vi "Cmag Move to (SubVI).vi"(9 "Instrument":T1 {"Input (1;B)" items=["A", "B"]; "Input (0:A) 325" items=["A", "B"]; "Input (0:A)" items=["A", "B"]; "Heater Output (1:1)" items=["1"=1, "2"=2]}, 10 "字符串":string) -> (0 "错误输出":errorcluster)   [LabVIEW 2019, in "Take Seq.lvlib"]
uses:
  Take Seq.lvlib
  ctl/Instrument.ctl
  <vilib>/NI/Modbus Library/API/Master/Modbus Master.lvclass
  ctl/Instrument Type.ctl
  lib/QDInstrument.dll
  ctl/335 state.ctl
  ctl/limit.ctl
  ctl/9T mag field stauts.ctl
  9T cmag.lvlib
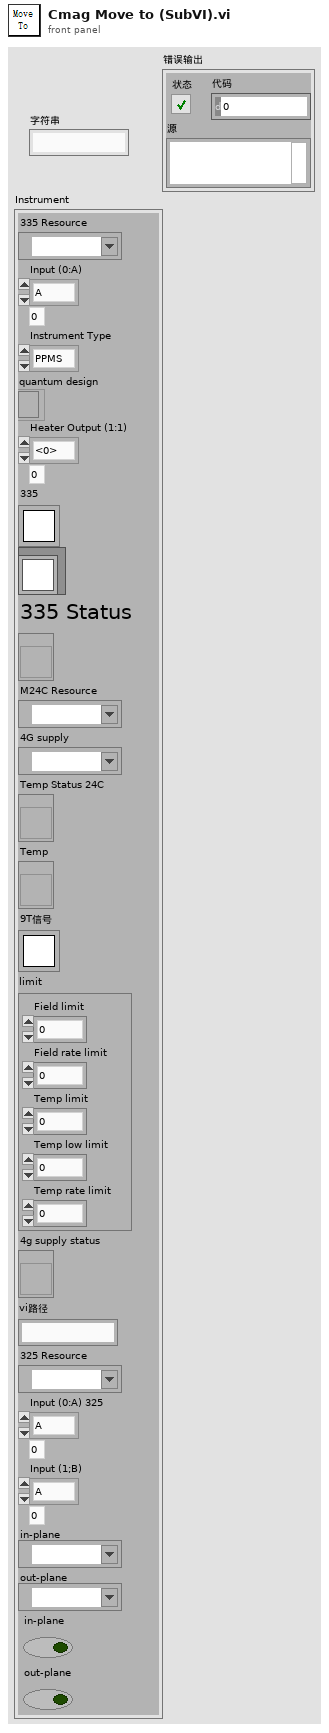
[diagram p1: front panel]
types:
  T1 = typedef "Instrument.ctl" = cluster{"335 Resource":refnum<visa-resource-name>, "Input (0:A)":u16, "Instrument Type":T2, "quantum design":refnum<k24>, "Heater Output (1:1)":u16, "semaphore":T3, "TCP master instance":refnum<class "Modbus Master.lvclass">, "335 Status":refnum<vi>, "M24C Resource":refnum<visa-resource-name>, "4G supply":refnum<visa-resource-name>, "Temp Status 24C":refnum<vi>, "Temp":refnum<vi>, "9T信号":T3, "limit":T4, "4g supply status":refnum<vi>, "vi路径":string, "325 Resource ":refnum<visa-resource-name>, "Input (0:A) 325":u16, "Input (1;B)":u16, "in-plane":refnum<visa-resource-name>, "out-plane":refnum<visa-resource-name>, "in-plane":bool, "out-plane":bool}
  T2 = typedef "Instrument Type.ctl" = enum16{"PPMS", "VersaLab", "DynaCool", "SVSM", "PPMS-Rotate", "Lakeshore335", "9T mag"}
  T3 = typedef "Semaphore RefNum" = refnum<k1>
  T4 = typedef "limit.ctl" = cluster{"Field limit":dbl, "Field rate limit":dbl, "Temp limit":dbl, "Temp low limit":dbl, "Temp rate limit ":dbl}
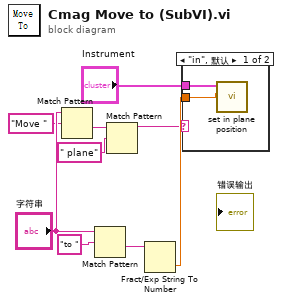
[diagram p0: block diagram]
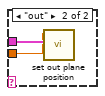
[diagram p2: hidden frame]
diagram:
  n1 = Match Pattern(string="字符串", regular expression="Move " ("正则表达式")) -> (after substring=w2:string)  [unwired: 1 in, 3 out]
  n2 = Match Pattern(string="字符串", regular expression="to " ("正则表达式")) -> (after substring=w9:string)  [unwired: 1 in, 3 out]
  n3 = Match Pattern(string=w2, regular expression=" plane" ("正则表达式")) -> (before substring=w1:string)  [unwired: 1 in, 3 out]
  n4 = Fract/Exp String To Number(string=w9) -> (number=w6:dbl)  [unwired: 3 in, 1 out]
  n5 = case shown="\"in\", 默认" w1 {
    tunnel: "Instrument" -> [w11 w13]
    tunnel: w6 -> [w10 w12]
    frame "in", Default {
      n6 = call "set in plane position.vi"("Value"=w10, "Instrument"=w11) -> ()  [unwired: 10 in]
    }
    frame "out" {
      n7 = call "set out plane position.vi"("Instrument"=w13, "Value"=w12) -> ()  [unwired: 10 in]
    }
  }
